vi "Variant to config data - Write.vi"(5 "Type":T1, 6 "Control in":refnum<vi>, 7 "Section Name":string, 8 "error in (no error)":errorcluster, 9 "Value":variant, 10 "Key Name":string, 11 "FIle refnum IN":T2) -> (0 "error out":errorcluster, 3 "Refnum out":T2)   [LabVIEW 2017]
uses:
  <vilib>/Utility/config.llb/Config Data RefNum.ctl
  <vilib>/Utility/Data Type/Type Definitions/Data Type.ctl
  <vilib>/Utility/config.llb/Write Key (String).vi
  <vilib>/Utility/config.llb/Write Key (Double).vi
  <vilib>/Utility/config.llb/Write Key (Boolean).vi
  <vilib>/Utility/config.llb/Write Key (I32).vi
  <vilib>/Utility/config.llb/Write Key (U32).vi
  <vilib>/Utility/config.llb/NI_LVConfig.lvlib
  <vilib>/Utility/Data Type/NI_Data Type.lvlib
panel:
  out "error out 2":errorcluster
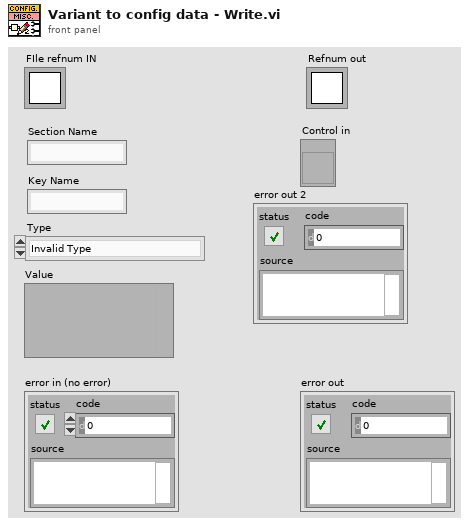
[diagram p1: front panel]
types:
  T1 = typedef "NI_Data Type.lvlib/Data Type.ctl" = enum8{"Invalid Type", "Void", "I8", "I16", "I32", "I64", "U8", "U16", "U32", "U64", "Single Float", "Double Float", "Extended Float", "Single Complex", "Double Complex", "Extended Complex", "Enum U8", "Enum U16", "Enum U32", "Enum U64", "Single Float With Unit", "Double Float With Unit", "Extended Float With Unit", "Single Complex with Unit", "Double Complex with Unit", "Extended Complex with Unit", "Boolean", "String", "Path", "Picture", "Tag", "Array", "Cluster", "Variant", "LV Variant", "Waveform", "Timestamp", "Digital Waveform", "Digital Data", "ExpressData", "Refnum", "External Data", "VI", "Poly VI", "LabVIEW Class Instance", "Fixed Point"}
  T2 = typedef "NI_LVConfig.lvlib/Config Data RefNum.ctl" = refnum<k1>
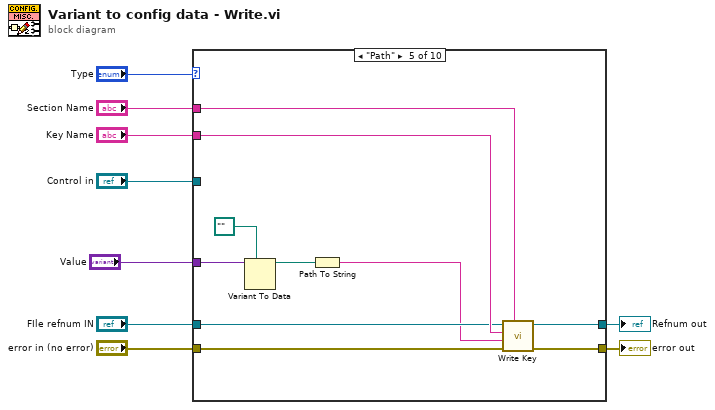
[diagram p0: block diagram]
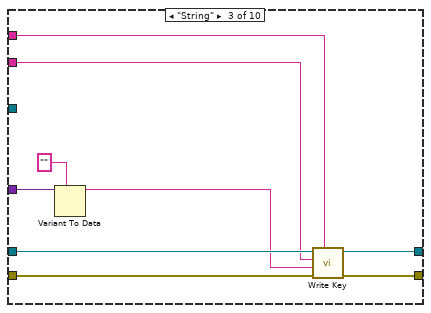
[diagram p4: hidden frame]
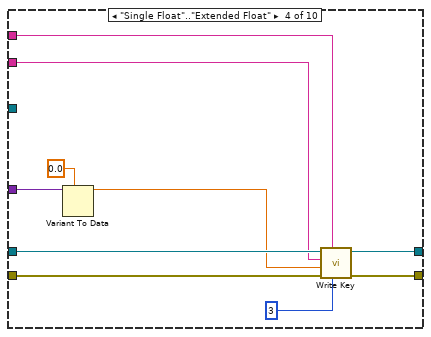
[diagram p5: hidden frame]
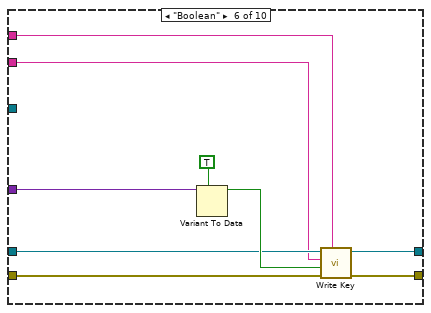
[diagram p6: hidden frame]
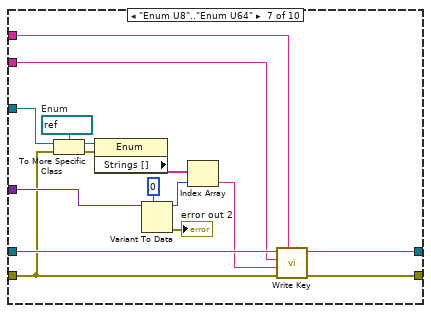
[diagram p7: hidden frame]
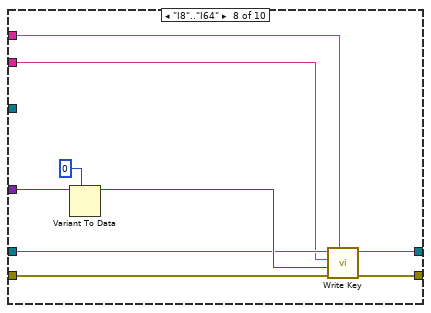
[diagram p8: hidden frame]
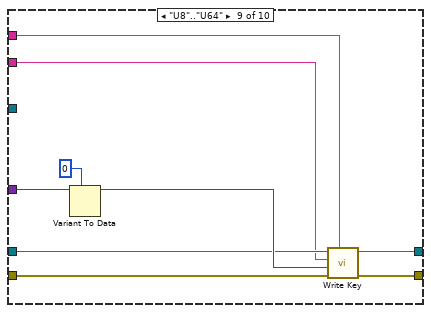
[diagram p9: hidden frame]
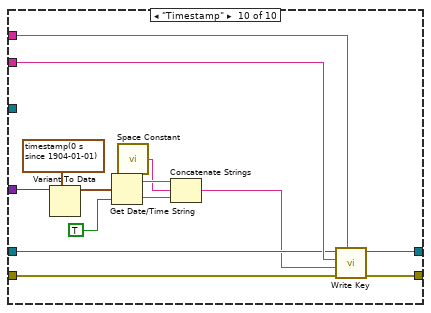
[diagram p10: hidden frame]
diagram:
  n1 = case shown="\"Path\"" "Type" {
    tunnel: "error in (no error)" -> [w10 w12 w22 w31 w38 w49 w57 w73 w82 w95]
    tunnel: "FIle refnum IN" -> [w11 w13 w21 w32 w39 w50 w58 w74 w83 w96]
    tunnel: "Section Name" -> [_ _ w20 w26 w42 w43 w55 w71 w80 w98]
    tunnel: "Key Name" -> [_ _ w19 w27 w41 w44 w54 w72 w81 w99]
    tunnel: "Value" -> [_ _ w18 w28 w40 w45 w60 w70 w79 w97]
    tunnel: [w11 w13 w15 w30 w37 w48 w59 w69 w78 w94] -> w7
    tunnel: [w10 w12 w14 w29 w36 w47 w56 w68 w77 w93] -> w8
    tunnel: "Control in" -> [_ _ _ _ _ _ w61 _ _ _]
    frame "Invalid Type", Default {
    }
    frame "Void" {
    }
    frame "String" {
      n2 = Variant To Data(type="", Variant=w18) -> (data=w16:string)  [unwired: 1 in, 1 out]
      n3 = call-poly <vilib>:"Write Key.vi"("section"=w20, "error in (no error)"=w22, "value"=w16, "key"=w19, "refnum"=w21) -> ("error out"=w14:errorcluster, "refnum out"=w15:T2)  [unwired: 4 in, 1 out]
    }
    frame "Single Float".."Extended Float" {
      n4 = Variant To Data(type=0.0, Variant=w28) -> (data=w24:dbl)  [unwired: 1 in, 1 out]
      n5 = call-poly <vilib>:"Write Key.vi"("precision (6)"=i16 3, "section"=w26, "error in (no error)"=w31, "value"=w24, "key"=w27, "refnum"=w32) -> ("error out"=w29:errorcluster, "refnum out"=w30:T2)  [unwired: 3 in, 1 out]
    }
    frame "Path" {
      n6 = Variant To Data(type=path "", Variant=w40) -> (data=w34:path)  [unwired: 1 in, 1 out]
      n7 = Path To String(path=w34) -> (string=w33:string)
      n8 = call-poly <vilib>:"Write Key.vi"("section"=w42, "error in (no error)"=w38, "value"=w33, "key"=w41, "refnum"=w39) -> ("error out"=w36:errorcluster, "refnum out"=w37:T2)  [unwired: 4 in, 1 out]
    }
    frame "Boolean" {
      n9 = Variant To Data(type=TRUE, Variant=w45) -> (data=w51:bool)  [unwired: 1 in, 1 out]
      n10 = call-poly <vilib>:"Write Key.vi"("section"=w43, "error in (no error)"=w49, "value"=w51, "key"=w44, "refnum"=w50) -> ("error out"=w47:errorcluster, "refnum out"=w48:T2)  [unwired: 4 in, 1 out]
    }
    frame "Enum U8".."Enum U64" {
      w67 = refnum<vi> refnum  # Enum
      n11 = To More Specific Class(target class=w67, reference=w61, error in=w57) -> (specific class reference=w65:refnum<vi>, error out=w66:errorcluster)
      n12 = property class="Enum"(reference=w65, error in=w66) -> ("Strings []"=w63:string[])  [unwired: 2 out]
      n13 = Variant To Data(type=0, Variant=w60) -> (data=w62:i32, error out=→"error out 2":errorcluster)  [unwired: 1 in]
      n14 = Index Array(array=w63, index=w62) -> (element=w53:string)
      n15 = call-poly <vilib>:"Write Key.vi"("section"=w55, "error in (no error)"=w57, "value"=w53, "key"=w54, "refnum"=w58) -> ("error out"=w56:errorcluster, "refnum out"=w59:T2)  [unwired: 4 in, 1 out]
    }
    frame "I8".."I64" {
      n16 = Variant To Data(type=0, Variant=w70) -> (data=w75:i32)  [unwired: 1 in, 1 out]
      n17 = call-poly <vilib>:"Write Key.vi"("section"=w71, "error in (no error)"=w73, "value"=w75, "key"=w72, "refnum"=w74) -> ("error out"=w68:errorcluster, "refnum out"=w69:T2)  [unwired: 4 in, 1 out]
    }
    frame "U8".."U64" {
      n18 = Variant To Data(type=u32 0, Variant=w79) -> (data=w84:u32)  [unwired: 1 in, 1 out]
      n19 = call-poly <vilib>:"Write Key.vi"("section"=w80, "error in (no error)"=w82, "value"=w84, "key"=w81, "refnum"=w83) -> ("error out"=w77:errorcluster, "refnum out"=w78:T2)  [unwired: 4 in, 1 out]
    }
    frame "Timestamp" {
      n20 = Variant To Data(type=timestamp(0 s since 1904-01-01), Variant=w97) -> (data=w91:timestamp)  [unwired: 1 in, 1 out]
      n21 = Get Date/Time String(seconds (now)=w91, want seconds? (F)=TRUE) -> (date string=w89:string, time string=w88:string)  [unwired: 1 in]
      n22 = call <vilib>:"Space Constant.vi"() -> ("String"=w87:string)
      n23 = Concatenate Strings(w89, w87, w88) -> (w86:string)
      n24 = call-poly <vilib>:"Write Key.vi"("section"=w98, "error in (no error)"=w95, "value"=w86, "key"=w99, "refnum"=w96) -> ("error out"=w93:errorcluster, "refnum out"=w94:T2)  [unwired: 4 in, 1 out]
    }
  }
  "error out" <- w8
  "Refnum out" <- w7
